vi "Test Method Result Has Test Name When Inheriting Test.vi"(8 "error in (no error)":errorcluster, 11 "Pass Assertion Test In":refnum<class "Method Result Test.lvclass">) -> (0 "error out":errorcluster, 3 "Pass Assertion Test Out":refnum<class "Method Result Test.lvclass">)   [LabVIEW 2020, in "LUnit Tests.lvlib" / "Method Result Test.lvclass"]
uses:
  Method Result Test.lvclass
  C:/Program Files (x86)/National Instruments/LabVIEW 2020/vi.lib/Astemes/LUnit/Test Case.lvclass
  Test Dummys/Descending Test Test Case/Descending Test Test Case.lvclass
  C:/Git/astemes-lunit/source/Framework/Test Case/LUnit Test Case.lvclass
  <vilib>/Astemes/LUnit/Test Case.lvclass/Test Case.ctl
  f6c42c16-fc45-4cfb-bf4c-3c6ef48240ea.vi
  1a9cf63c-f8e3-48b5-90d4-a0169b03c261.vi
  <vilib>/Astemes/LUnit/Palette/Pass.vi
  <vilib>/Astemes/LUnit/Palette/Fail.vi
  <vilib>/Astemes/LUnit/Compare Variants.vi
  <vilib>/Astemes/LUnit/Describe Comparison.vi
  <vilib>/Astemes/LUnit/Set Assertion Type.vi
  <vilib>/Astemes/LUnit/Add test result.vi
  <vilib>/Astemes/LUnit/Variant to string.vi
  <vilib>/Astemes/LUnit/LUnit Record Assertion Result.vi
  <vilib>/Astemes/LUnit/LUnit Aggregate Assertion Results.vi
  <vilib>/Astemes/LUnit/Method Result/LUnit Merge Status.vi
  <vilib>/Astemes/LUnit/LUnit Concatenate result strings.vi
  <vilib>/Utility/Data Type/Get Type Information.vi
  <vilib>/Utility/LVClass/Get LV Class Name.vi
  Method Result Test.lvclass/Method Result Test.ctl
  source/Framework/Execution API/Execution API.lvclass
  C:/Git/astemes-lunit/tests/Test Dummys/Test Test Case/Test Test Case.lvclass
  C:/Git/astemes-lunit/tests/Test Dummys/Descending Test Test Case/Descending Test Test Case.lvclass
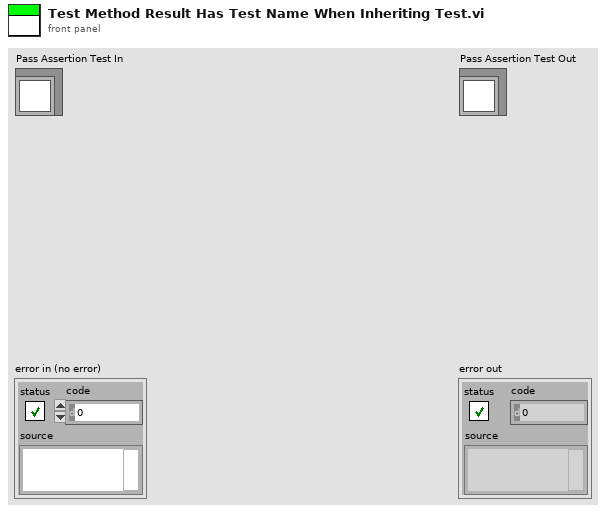
[diagram p1: front panel]
types:
  T1 = cluster{"Result Events":refnum<event-registration>, "Event Registration Refnum":refnum<event-registration>}
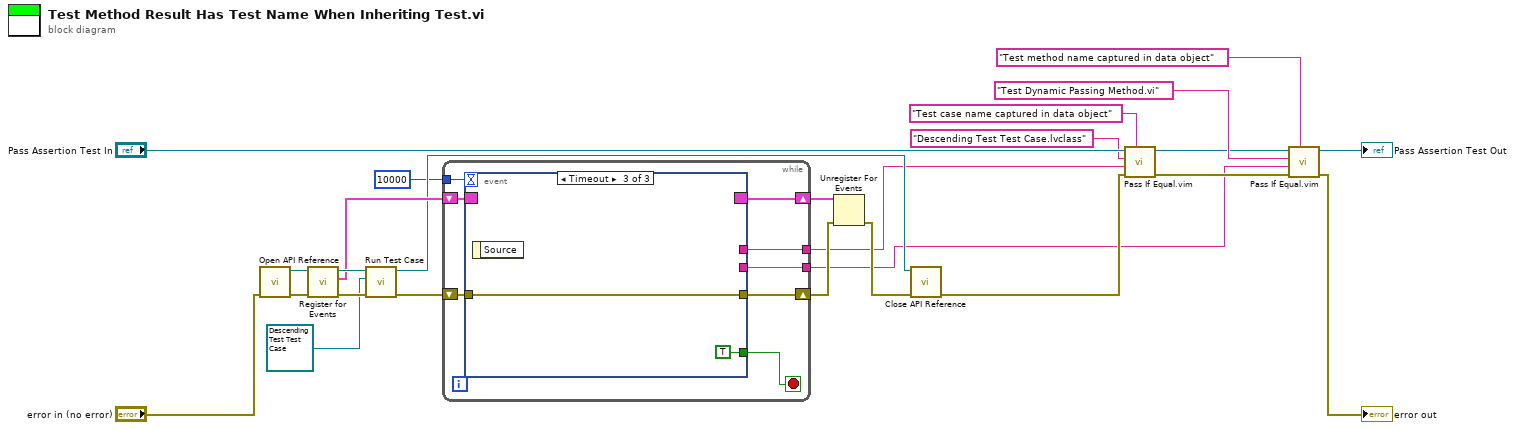
[diagram p0: block diagram]
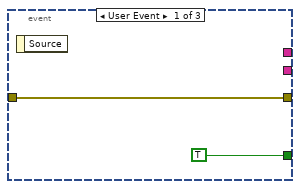
[diagram p2: hidden frame]
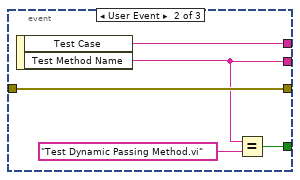
[diagram p3: hidden frame]
diagram:
  n1 = call "Open API Reference.vi"("error in (no error)"="error in (no error)") -> ("error out"=w24:errorcluster, "Execution API out"=w25:refnum<class "Execution API.lvclass">)  [unwired: 9 in]
  n2 = call "Register for Events.vi"("error in (no error)"=w24, "Execution API in"=w25) -> ("error out"=w22:errorcluster, "Event Registrations"=w21:T1, "Execution API out"=w23:refnum<class "Execution API.lvclass">)  [unwired: 7 in]
  n3 = call "Run Test Case.vi"("error in (no error)"=w22, "Test Case"=refnum<class "Descending Test Test Case.lvclass"> refnum ("Framework Tests.lvlib:Descending Test Test Case.lvclass"), "Execution API In"=w23) -> ("error out"=w18:errorcluster, "Execution API Out"=w11:refnum<class "Execution API.lvclass">)  [unwired: 7 in]
  n4 = while {
    shift-right: [w32] -> w20
    shift-left: w21 -> [w33]
    shift-right: [w30] -> w17
    shift-left: w18 -> [w31]
    tunnel: [w28] -> w3
    tunnel: [w27] -> w2
    tunnel: 10000 -> [w26]
    stop <- w29 stop-if-true
    n5 = event shown="[2] Timeout" {
      selector: w33 -> [_ _ _]
      dyn-events: [_ _ _] -> w32
      timeout: w26 -> [_ _ _]
      tunnel: w31 -> [w35 w38 w42]
      tunnel: [w35 w38 w42] -> w30
      tunnel: [TRUE w39 TRUE] -> w29
      tunnel: [_ w37 _] -> w28
      tunnel: [_ w36 _] -> w27
      event User Event {
        n6 = event-data() -> ()  [unwired: 1 in, 1 out]
      }
      event User Event {
        n7 = event-data() -> ("Test Case"=w37:string, "Test Method Name"=w36:string)  [unwired: 1 in]
        n8 = Equal?(x=w36, y="Test Dynamic Passing Method.vi") -> (x = y?=w39:bool)
      }
      event Timeout {
        n9 = event-data() -> ()  [unwired: 1 in, 1 out]
      }
    }
  }
  n10 = Unregister For Events(event registration refnum=w20, error in=w17) -> (error out=w16:errorcluster)
  n11 = call "Close API Reference.vi"("error in (no error)"=w16, "Execution API in"=w11) -> ("error out"=w7:errorcluster)  [unwired: 9 in]
  n12 = call "Pass If Equal.vim"("Description"="Test case name captured in data object", "error in (no error)"=w7, "Actual"=w3, "Expected"="Descending Test Test Case.lvclass", "LUnit Test Case In"="Pass Assertion Test In") -> ("error out"=w6:errorcluster, "LUnit Test Case Out"=w8:refnum<class "Method Result Test.lvclass">)  [unwired: 5 in]
  n13 = call "Pass If Equal.vim"("Description"="Test method name captured in data object", "error in (no error)"=w6, "Actual"=w2, "Expected"="Test Dynamic Passing Method.vi", "LUnit Test Case In"=w8) -> ("error out"=→"error out":errorcluster, "LUnit Test Case Out"=→"Pass Assertion Test Out":refnum<class "Method Result Test.lvclass">)  [unwired: 5 in]
